vi "RelayController.vi"() -> ()   [LabVIEW 2016]
uses:
  <vilib>/Utility/miscctls.llb/LVRowAndColumnTypeDef.ctl
  <vilib>/Utility/file.llb/Read Delimited Spreadsheet (string).vi
  <vilib>/Utility/file.llb/Write Delimited Spreadsheet (string).vi
panel:
  out "running?":bool
  out "Controller OK?":bool
  out "countdown":dbl
  in  "resolution (ms)":u32=100 min=100 max=1000
  out "relay message":string
  in  "Port Name":refnum<visa-resource-name>
  in  "save sequence":bool
  in  "start seq":bool
  in  "Delete":bool
  in  "Insert":bool
  in  "Duration (s)":dbl=30.0
  in  "Set to OFF #":string
  in  "Set to ON #":string
  in  "Seq#":u32
  out "Sequence list":string[][](table)
  in  "load sequence":bool
  out "Current time":timestamp format="%<%.3X %x>T"
  out "Relay 24-31":bool[](array[boolean])
  out "Relay 8-15":bool[](array[boolean])
  out "Relay 16-23":bool[](array[boolean])
  in  "quit":bool
  in  "Typical duration (s)":dbl=30.0 min=0.0
  out "Relay 0-7":bool[](array[boolean])
  # "0"
  # "1"
  # "2"
  # "3"
  # "4"
  # "5"
  # "6"
  # "7"
  # "8"
  # "9"
  # "10"
  # "11"
  # "12"
  # "13"
  # "14"
  # "15"
  # "16"
  # "17"
  # "18"
  # "19"
  # "20"
  # "21"
  # "22"
  # "23"
  # "24"
  # "25"
  # "26"
  # "27"
  # "28"
  # "29"
  # "30"
  # "31"
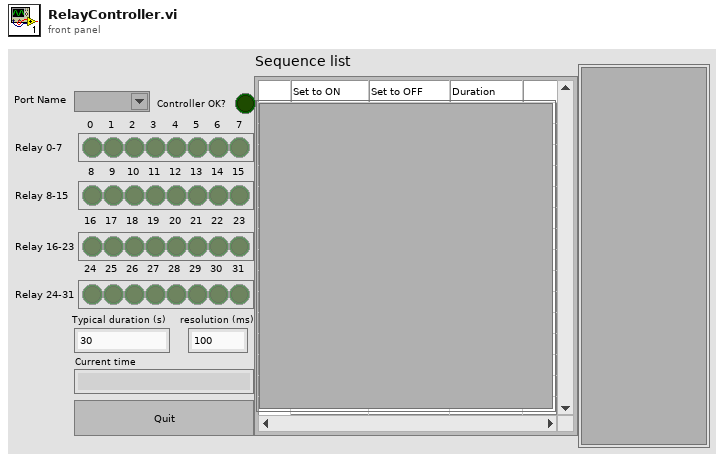
[diagram p1: front panel]
types:
  T1 = enum8{"Enabled", "Disabled", "Disabled and Grayed Out"}
  T2 = cluster{"Set to ON":string, "Set to OFF":string, "Duration (s)":dbl}[]
  T3 = cluster{"baud rate (9600)":u32, "data bits (8)":u16, "stop bits (10: 1 bit)":u16, "parity (0:none)":enum16{"None", "Odd", "Even", "Mark", "Space"}, "flow control (0:none)":u16, "timeout (10sec)":u32, "Enable Termination\nChar (T)":bool, "termination char\n(0xA = '\\n' = LF)\n(0xD = '\\r' = CF) ":u8}
  T4 = typedef "LVRowAndColumnTypeDef.ctl" = cluster{"Row":i32, "Column":i32}
  T5 = cluster{"Set to ON":string, "Set to OFF":string, "Duration (s)":dbl}
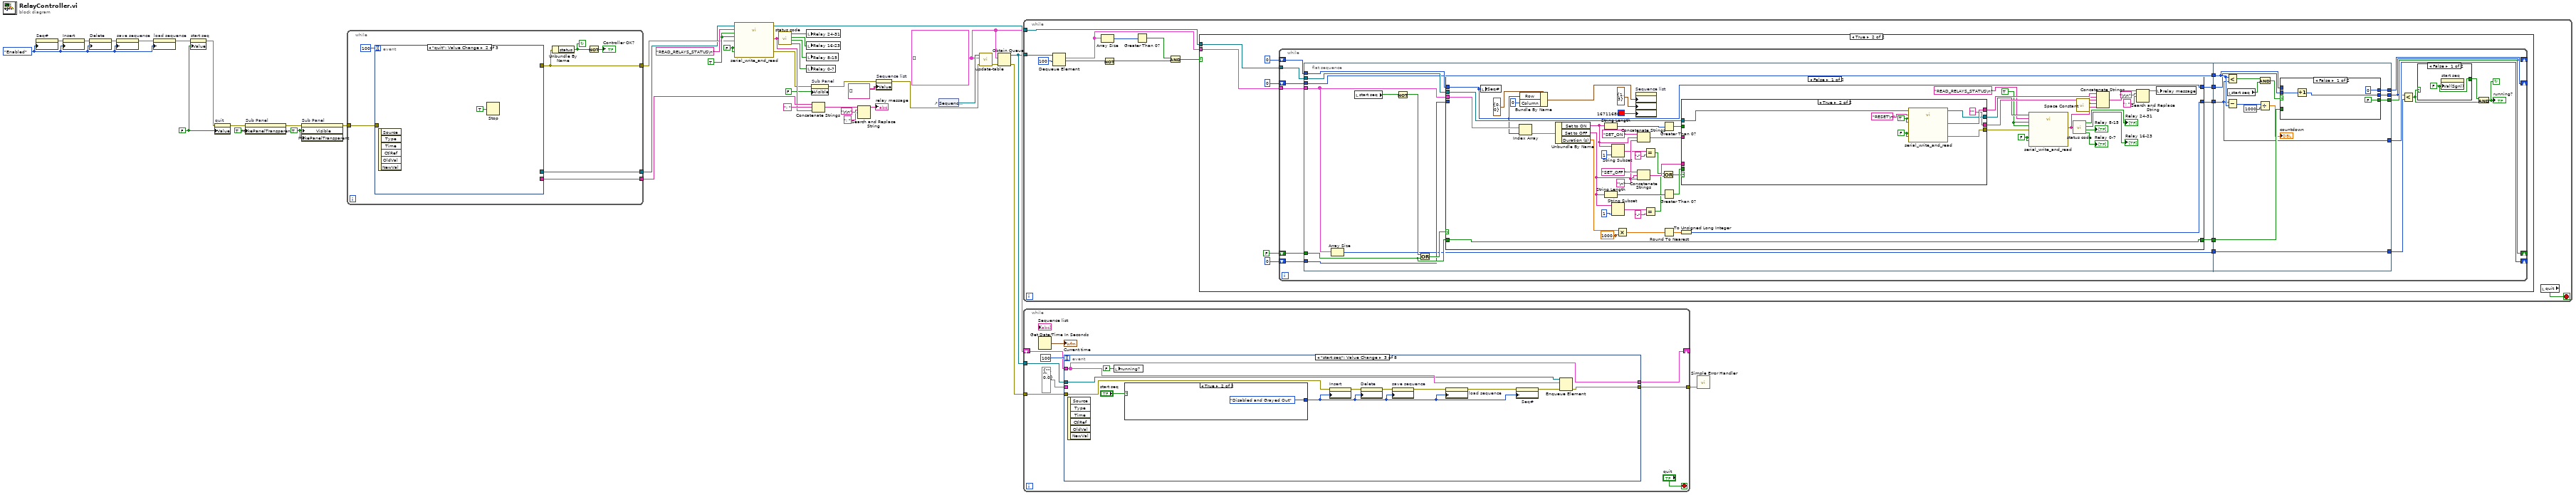
[diagram p0: block diagram]
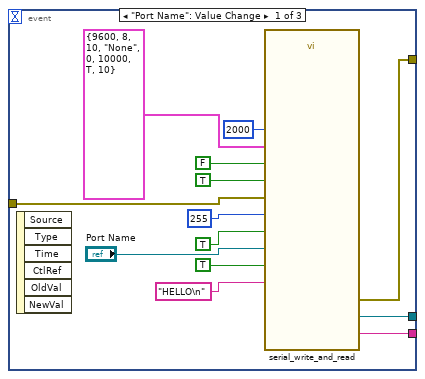
[diagram p2: hidden frame]
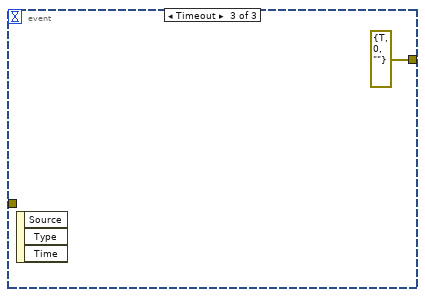
[diagram p3: hidden frame]
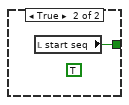
[diagram p5: hidden frame]
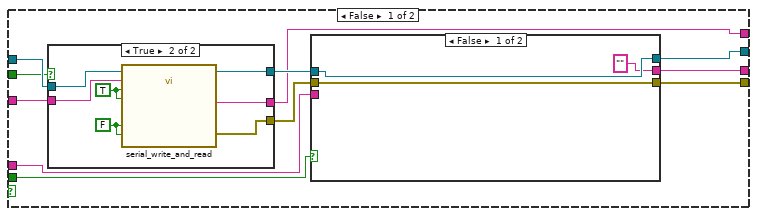
[diagram p6: hidden frame]
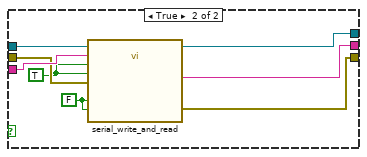
[diagram p7: hidden frame]
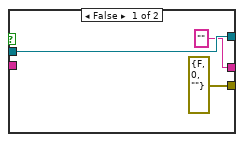
[diagram p8: hidden frame]
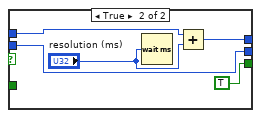
[diagram p10: hidden frame]
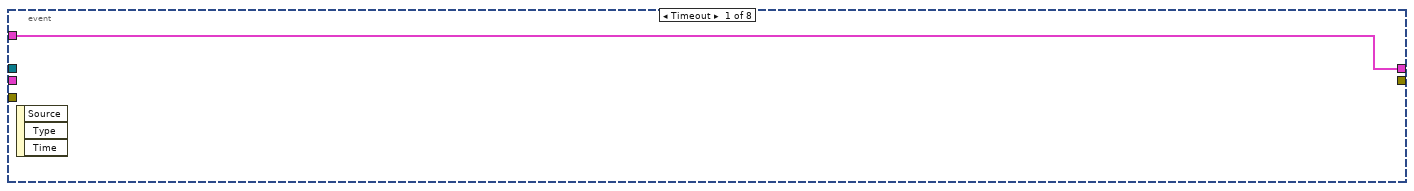
[diagram p11: hidden frame]
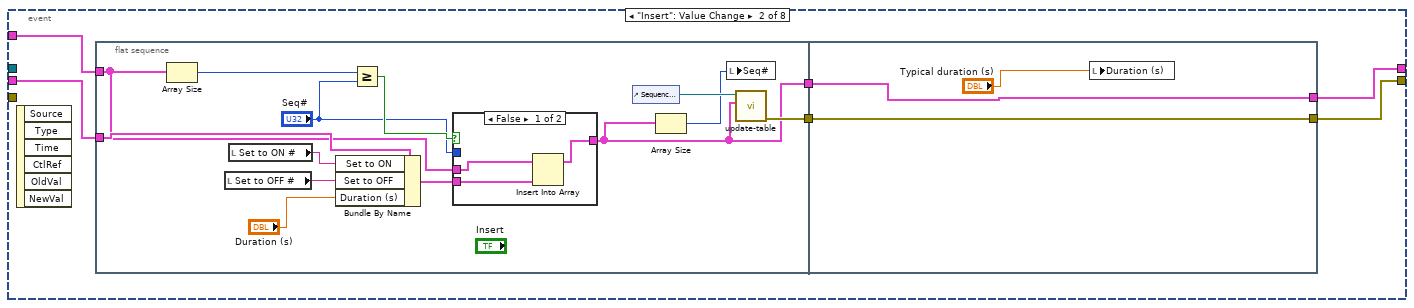
[diagram p12: hidden frame]
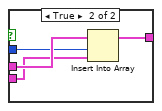
[diagram p13: hidden frame]
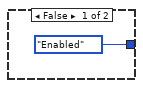
[diagram p14: hidden frame]
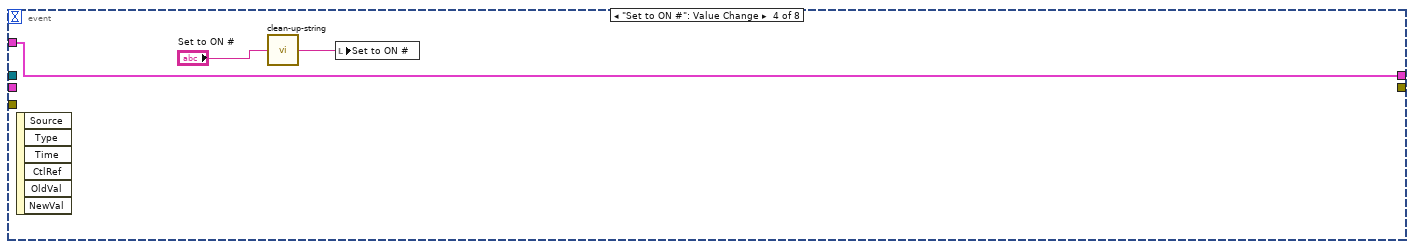
[diagram p15: hidden frame]
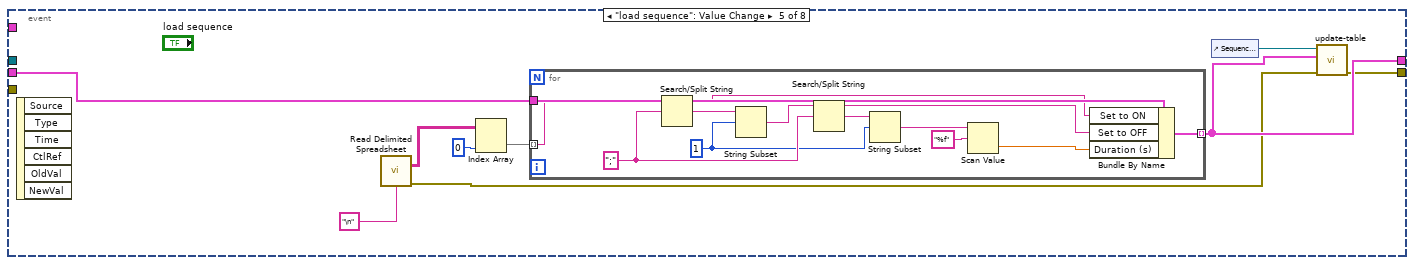
[diagram p16: hidden frame]
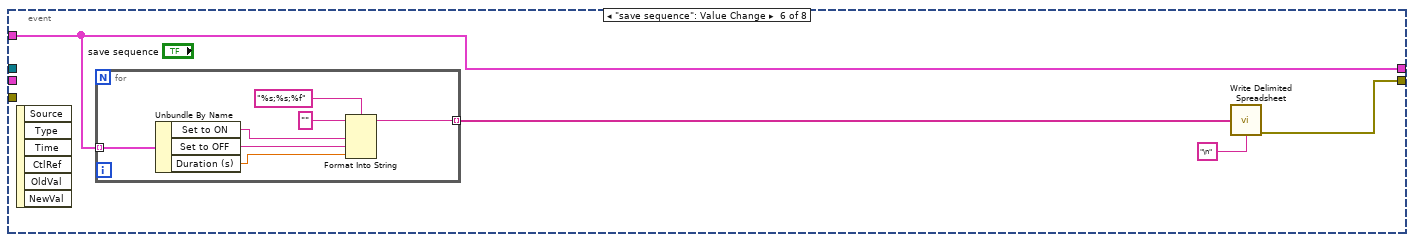
[diagram p17: hidden frame]
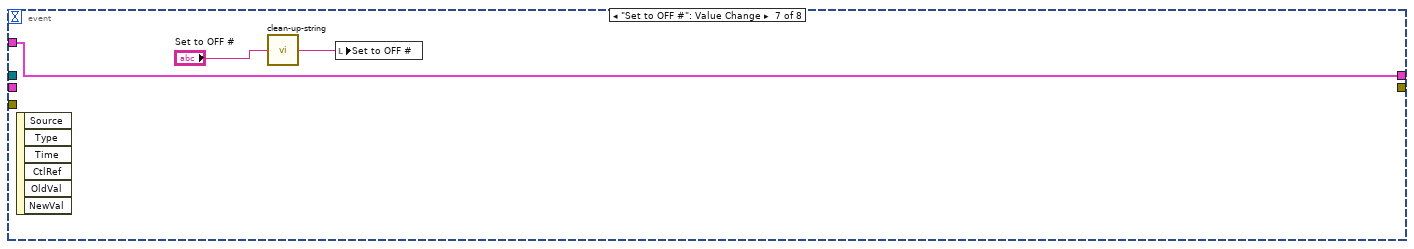
[diagram p18: hidden frame]
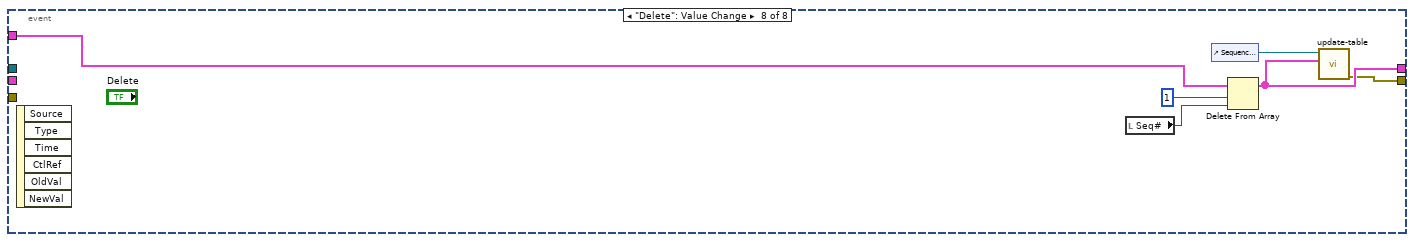
[diagram p19: hidden frame]
diagram:
  w6 = TRUE ("Visible")
  w27 = FALSE ("reconnect?")
  w28 = TRUE
  w13 = T1."Enabled" ("Disabled")
  w34 = FALSE ("start seq")
  w37 = T2 []
  n1 = property on="Seq#" class="DigNum (strict)"("DisabledEnum"=w13) -> (error out=w14:errorcluster)  [unwired: 2 in, 1 out]
  n2 = property on="Insert" class="Bool"(error in=w14, "DisabledEnum"=w13) -> (error out=w33:errorcluster)  [unwired: 1 in, 1 out]
  n3 = property on="Delete" class="Bool"(error in=w33, "DisabledEnum"=w13) -> (error out=w32:errorcluster)  [unwired: 1 in, 1 out]
  n4 = property on="save sequence" class="Bool"(error in=w32, "DisabledEnum"=w13) -> (error out=w31:errorcluster)  [unwired: 1 in, 1 out]
  n5 = property on="load sequence" class="Bool"(error in=w31, "DisabledEnum"=w13) -> (error out=w30:errorcluster)  [unwired: 1 in, 1 out]
  n6 = property on="start seq" class="Bool (strict)"(error in=w30, "Value"=w34) -> (error out=w35:errorcluster)  [unwired: 1 in, 1 out]
  n7 = property on="quit" class="Bool (strict)"(error in=w35, "Value"=w34) -> (error out=w12:errorcluster)  [unwired: 1 in, 1 out]
  n8 = property on="Sub Panel" class="SubPnl"(error in=w12, "MakePanelTransparent"=TRUE ("Panel Transparent")) -> (error out=w5:errorcluster)  [unwired: 1 in, 1 out]
  n9 = property on="Sub Panel" class="SubPnl"(error in=w5, "Visible"=w6, "MakePanelTransparent"=w6) -> (error out=w4:errorcluster)  [unwired: 1 in, 1 out]
  n10 = while {
    tunnel: [w48] -> w8
    tunnel: [w47] -> w23
    tunnel: w4 -> [w46]
    tunnel: [w45] -> w24
    stop <- w43 continue-if-true
    n11 = event shown="[1] \"quit\": Value Change" {
      selector: _ -> [_ _ _]
      dyn-events: _ -> [_ _ _]
      timeout: 100 -> [_ _ _]
      tunnel: [w54 _ _] -> w48
      tunnel: w46 -> [w51 _ _]
      tunnel: [w50 _ errorcluster {"status"=TRUE, "code"=0, "source"=""} ("error out")] -> w45
      tunnel: [w49 _ _] -> w47
      event "Port Name": Value Change {
        n12 = event-data() -> ()  [unwired: 1 in, 6 out]
        n13 = call "serial_write_and_read.vi"("port name in"="Port Name", "reconnect?"=TRUE, "disconnect?"=FALSE, "write buffer"="HELLO\n", "do writing?"=TRUE, "expecting response?"=TRUE, "error in"=w51, "expected max length"=u32 255, "connection parameters"=T3 {"baud rate (9600)"=9600, "data bits (8)"=8, "stop bits (10: 1 bit)"=10, "parity (0:none)"=enum."None", "flow control (0:none)"=0, "timeout (10sec)"=10000, "Enable Termination\nChar (T)"=TRUE, "termination char\n(0xA = '\\n' = LF)\n(0xD = '\\r' = CF) "=10}, "COM response delay"=u32 2000) -> ("port name out"=w54:refnum<visa-resource-name>, "read buffer"=w49:string, "error out"=w50:errorcluster)  [unwired: 3 in]
      }
      event "quit": Value Change {
        n14 = event-data() -> ()  [unwired: 1 in, 6 out]
        n15 = Stop(stop? (T)=TRUE) -> ()
      }
      event Timeout {
        n16 = event-data() -> ()  [unwired: 1 in, 3 out]
      }
    }
    n17 = Unbundle By Name(w45) -> ("status"=w43:bool)
    n18 = Not(x=w43) -> (.not. x?=→"Controller OK?":bool)
  }
  n19 = call "serial_write_and_read.vi"("port name in"=w8, "reconnect?"=w27, "disconnect?"=w27, "write buffer"="READ_RELAYS_STATUS\n", "do writing?"=w28, "expecting response?"=w28, "error in"=w24) -> ("port name out"=w7:refnum<visa-resource-name>, "read buffer"=w21:string, "error out"=w3:errorcluster)  [unwired: 6 in]
  n20 = call "status code.vi"("status code"=w21) -> ("Relay 24-31"=w15:bool[], "Relay 16-23"=w16:bool[], "Relay 8-15"=w17:bool[], "Relay 0-7"=w18:bool[])
  n21 = local write "Relay 24-31"(w15) -> ()
  n22 = local write "Relay 16-23"(w16) -> ()
  n23 = local write "Relay 8-15"(w17) -> ()
  n24 = local write "Relay 0-7"(w18) -> ()
  n25 = property on="Sub Panel" class="SubPnl"(error in=w3, "Visible"=FALSE) -> (error out=w2:errorcluster)  [unwired: 1 in, 1 out]
  n26 = Concatenate Strings(w23, "; " ("string"), w21) -> (w20:string)
  n27 = Search and Replace String(input string=w20, search string="\r\n", replace string="; " ("replace string (\"\")")) -> (result string=→"relay message":string)  [unwired: 5 in, 3 out]
  n28 = property on="Sequence list" class="Tbl (strict)"(error in=w2, "Value"=string[][] []) -> (error out=w11:errorcluster)  [unwired: 1 in, 1 out]
  n29 = control-ref of="Sequence list"() -> (w39:refnum<vi>)
  n30 = call "update-table.vi"("error in (no error)"=w11, "contents"=w37, "Table ref in"=w39) -> ("error out"=w10:errorcluster)  [unwired: 3 in, 1 out]
  n31 = Obtain Queue(element data type=w37, error in (no error)=w10) -> (queue out=w36:refnum<queue>, error out=w9:errorcluster)  [unwired: 3 in, 1 out]
  n32 = while {
    tunnel: w36 -> [w73]
    tunnel: w7 -> [w65]
    stop <- w64 stop-if-true
    n33 = Dequeue Element(queue=w73, timeout in ms (-1)=100) -> (element=w71:T2, timed out?=w69:bool)  [unwired: 1 in, 2 out]
    n34 = Array Size(array=w71) -> (size(s)=w70:i32)
    n35 = Not(x=w69) -> (.not. x?=w67:bool)
    n36 = Greater Than 0?(x=w70) -> (x > 0?=w68:bool)
    n37 = And(x=w68, y=w67) -> (x .and. y?=w66:bool)
    n38 = case shown="True" w66 {
      tunnel: w71 -> [_ w79]
      tunnel: w65 -> [_ w75]
      frame False {
      }
      frame True {
        n39 = while {
          tunnel: w79 -> [w90]
          shift-right: [w93] -> _
          shift-left: u32 0 -> [w87]
          shift-right: [w81] -> _
          shift-left: 0 -> [w82]
          shift-right: [w96] -> _
          shift-left: FALSE -> [w98]
          tunnel: w75 -> [w97]
          shift-right: [w83] -> _
          shift-left: u32 0 -> [w89]
          stop <- w80 continue-if-true
          n40 = flat-sequence {
            tunnel: w98 -> [w107]
            tunnel: w97 -> [w113]
            tunnel: w82 -> [w106]
            tunnel: [w112] -> w95
            tunnel: [w111] -> w94
            tunnel: w90 -> [w101]
            tunnel: w89 -> [w104]
            tunnel: [w105] -> w88
            tunnel: w87 -> [w103]
            tunnel: [w103] -> w86
            tunnel: [w102] -> w85
            tunnel: [w209] -> w81
            tunnel: [w217] -> w96
            tunnel: w95 -> [w218]
            tunnel: w94 -> [w210]
            tunnel: [w222] -> w93
            tunnel: w88 -> [w211]
            tunnel: w86 -> [w213]
            tunnel: w85 -> [w212]
            tunnel: [w212] -> w84
            tunnel: [w211] -> w83
            frame #0 {
              n41 = Array Size(array=w101) -> (size(s)=w102:i32)
              n42 = local read "start seq"() -> (w110:bool)
              n43 = Not(x=w110) -> (.not. x?=w109:bool)
              n44 = Or(x=w109, y=w107) -> (x .or. y?=w108:bool)
              n45 = case shown="False" w108 {
                tunnel: w113 -> [w165 _]
                tunnel: [w133 w207] -> w112
                tunnel: w106 -> [w114 w208]
                tunnel: [w114 w208] -> w111
                tunnel: w107 -> [w133 w207]
                tunnel: [w119 w206] -> w105
                tunnel: w104 -> [_ w206]
                tunnel: w101 -> [w122 _]
                frame False {
                  w134 = FALSE ("reconnect?")
                  w135 = TRUE
                  w150 = "\n" ("string")
                  n46 = local write "Seq#"(w114) -> ()
                  n47 = Index Array(array=w122, index=w114) -> (element=w127:T5)
                  n48 = Bundle By Name(cluster=T4 {"Row"=0, "Column"=0} ("Selection Start"), "Row"=w114, "Column"=0) -> (w131:T4)
                  n49 = Unbundle By Name(w127) -> ("Set to ON"=w121:string, "Set to OFF"=w120:string, "Duration (s)"=w126:dbl)
                  n50 = String Length(string=w121) -> (length=w148:i32)
                  n51 = String Length(string=w120) -> (length=w147:i32)
                  n52 = String Subset(string=w121, length (rest)=1 ("length (rest)")) -> (substring=w142:string)  [unwired: 1 in]
                  n53 = String Subset(string=w120, length (rest)=1 ("length (rest)")) -> (substring=w139:string)  [unwired: 1 in]
                  n54 = Multiply(x=w126, y=1000.0) -> (x*y=w124:dbl)
                  n55 = property on="Sequence list" class="Tbl (strict)"("Selection Start"=w131, "Selection Size"=T4 {"Row"=1, "Column"=3}, "Selection Color"=u32 16711680) -> ()  [unwired: 2 in, 2 out]
                  n56 = Concatenate Strings("SET_ON " ("string"), w121, w150) -> (w163:string)
                  n57 = Concatenate Strings("SET_OFF " ("string"), w120, w150) -> (w161:string)
                  n58 = Equal?(x=w142, y="-") -> (x = y?=w138:bool)
                  n59 = Equal?(x=w139, y="-") -> (x = y?=w137:bool)
                  n60 = Or(x=w138, y=w137) -> (x .or. y?=w136:bool)
                  n61 = Greater Than 0?(x=w148) -> (x > 0?=w146:bool)
                  n62 = Greater Than 0?(x=w147) -> (x > 0?=w145:bool)
                  n63 = Round To Nearest(number=w124) -> (nearest integer value=w123:dbl)
                  n64 = To Unsigned Long Integer(number=w123) -> (unsigned 32bit integer=w119:u32)
                  n65 = case shown="True" w136 {
                    tunnel: w165 -> [w176 w204]
                    tunnel: w163 -> [w175 _]
                    tunnel: w161 -> [w174 _]
                    tunnel: [w172 w203] -> w160
                    tunnel: [w171 "" ("read buffer")] -> w159
                    tunnel: [w170 w200] -> w157
                    tunnel: [w168 w199] -> w149
                    tunnel: w146 -> [w167 _]
                    tunnel: w145 -> [w166 _]
                    frame False {
                      n66 = case shown="True" w167 {
                        tunnel: w176 -> [w190 w197]
                        tunnel: w175 -> [_ w196]
                        tunnel: [w190 w195] -> w173
                        tunnel: ["" ("read buffer") w194] -> w172
                        tunnel: [errorcluster {"status"=FALSE, "code"=0, "source"=""} ("error out") w193] -> w169
                        frame False {
                        }
                        frame True {
                          w191 = FALSE ("reconnect?")
                          w192 = TRUE ("do writing?")
                          n67 = call "serial_write_and_read.vi"("port name in"=w197, "reconnect?"=w191, "disconnect?"=w191, "write buffer"=w196, "do writing?"=w192, "expecting response?"=w192) -> ("port name out"=w195:refnum<visa-resource-name>, "read buffer"=w194:string, "error out"=w193:errorcluster)  [unwired: 7 in]
                        }
                      }
                      n68 = case shown="False" w166 {
                        tunnel: w174 -> [_ w187]
                        tunnel: w173 -> [w179 w186]
                        tunnel: ["" ("read buffer") w185] -> w171
                        tunnel: [w179 w184] -> w170
                        tunnel: w169 -> [w177 w183]
                        tunnel: [w177 w182] -> w168
                        frame False {
                        }
                        frame True {
                          w180 = FALSE ("reconnect?")
                          w181 = TRUE
                          n69 = call "serial_write_and_read.vi"("port name in"=w186, "reconnect?"=w180, "disconnect?"=w180, "write buffer"=w187, "do writing?"=w181, "expecting response?"=w181, "error in"=w183) -> ("port name out"=w184:refnum<visa-resource-name>, "read buffer"=w185:string, "error out"=w182:errorcluster)  [unwired: 6 in]
                        }
                      }
                    }
                    frame True {
                      w201 = TRUE ("do writing?")
                      w202 = FALSE ("reconnect?")
                      n70 = call "serial_write_and_read.vi"("port name in"=w204, "reconnect?"=w202, "disconnect?"=w202, "write buffer"="RESET\n", "do writing?"=w201, "expecting response?"=w201) -> ("port name out"=w200:refnum<visa-resource-name>, "read buffer"=w203:string, "error out"=w199:errorcluster)  [unwired: 7 in]
                    }
                  }
                  n71 = call "serial_write_and_read.vi"("port name in"=w157, "reconnect?"=w134, "disconnect?"=w134, "write buffer"="READ_RELAYS_STATUS\n", "do writing?"=w135, "expecting response?"=w135, "error in"=w149) -> ("read buffer"=w155:string)  [unwired: 6 in, 2 out]
                  n72 = call "status code.vi"("status code"=w155) -> ("Relay 24-31"=→"Relay 24-31":bool[], "Relay 16-23"=→"Relay 16-23":bool[], "Relay 8-15"=→"Relay 8-15":bool[], "Relay 0-7"=→"Relay 0-7":bool[])
                  n73 = call <vilib>:"Space Constant.vi"() -> ("String"=w158:string)
                  n74 = Concatenate Strings(w160, w158, w159, w158, w155) -> (w118:string)
                  n75 = Search and Replace String(input string=w118, search string="\r\n", replace string="; " ("replace string (\"\")")) -> (result string=w115:string)  [unwired: 5 in, 3 out]
                  n76 = local write "relay message"(w115) -> ()
                }
                frame True {
                }
              }
            }
            frame #1 {
              n77 = Less?(x=w213, y=w211) -> (x < y?=w220:bool)
              n78 = Subtract(x=w211, y=w213) -> (x-y=w216:u32)
              n79 = local read "start seq"() -> (w221:bool)
              n80 = Divide(x=w216, y=u32 1000) -> (x/y=→"countdown":dbl)
              n81 = And(x=w220, y=w221) -> (x .and. y?=w219:bool)
              n82 = case shown="False" w219 {
                tunnel: w213 -> [_ w231]
                tunnel: [u32 0 w230] -> w222
                tunnel: w218 -> [_ _]
                tunnel: [FALSE ("do writing?") TRUE ("do writing?")] -> w217
                tunnel: w210 -> [w224 w227]
                tunnel: [w223 w227] -> w209
                frame False {
                  n83 = Increment(x=w224) -> (x+1=w223:i32)
                }
                frame True {
                  n84 = Wait (ms)(milliseconds to wait="resolution (ms)") -> ()  [unwired: 1 out]
                  n85 = Add(x=w231, y="resolution (ms)") -> (x+y=w230:u32)
                }
              }
            }
          }
          n86 = Less?(x=w81, y=w84) -> (x < y?=w92:bool)
          n87 = case shown="False" w92 {
            tunnel: [w99 w100] -> w91
            frame False {
              w99 = FALSE ("start seq")
              n88 = property on="start seq" class="Bool (strict)"("Val(Sgnl)"=w99) -> ()  [unwired: 2 in, 2 out]
            }
            frame True {
              (unwired) TRUE ("running?")
              n89 = local read "start seq"() -> (w100:bool)
            }
          }
          n90 = And(x=w91, y=w92) -> (x .and. y?=w80:bool)
          "running?" <- w80
        }
      }
    }
    n91 = local read "quit"() -> (w64:bool)
  }
  n92 = while {
    shift-right: [w236] -> _
    shift-left: w37 -> [w238]
    tunnel: [w234] -> w40
    tunnel: w9 -> [w233]
    tunnel: w36 -> [w232]
    stop <- "quit" stop-if-true
    n93 = Get Date/Time In Seconds() -> (seconds since 1Jan1904=→"Current time":timestamp)
    n94 = event shown="[2] \"start seq\": Value Change" {
      selector: _ -> [_ _ _ _ _ _ _ _]
      dyn-events: _ -> [_ _ _ _ _ _ _ _]
      timeout: 100 -> [_ _ _ _ _ _ _ _]
      tunnel: w238 -> [w241 w246 w277 w285 _ w313 w321 w329]
      tunnel: T5 {"Set to ON"="", "Set to OFF"="", "Duration (s)"=0.0} ("element") -> [_ w247 _ _ w296 _ _ _]
      tunnel: [w241 w244 w277 w285 w290 w313 w321 w326] -> w236
      tunnel: [_ w245 w275 _ w289 w310 _ w324] -> w234
      tunnel: w233 -> [_ _ w281 _ _ _ _ _]
      tunnel: w232 -> [_ _ w276 _ _ _ _ _]
      event Timeout {
        n95 = event-data() -> ()  [unwired: 1 in, 3 out]
      }
      event "Insert": Value Change {
        n96 = event-data() -> ()  [unwired: 1 in, 6 out]
        n97 = flat-sequence {
          tunnel: w247 -> [w260]
          tunnel: w246 -> [w253]
          tunnel: [w250] -> w243
          tunnel: [w249] -> w242
          tunnel: [w269] -> w244
          tunnel: [w270] -> w245
          tunnel: w243 -> [w270]
          tunnel: w242 -> [w269]
          frame #0 {
            n98 = Array Size(array=w253) -> (size(s)=w255:i32)
            n99 = local read "Set to OFF #"() -> (w258:string)
            n100 = local read "Set to ON #"() -> (w259:string)
            n101 = Bundle By Name(cluster=w260, "Set to ON"=w259, "Set to OFF"=w258, "Duration (s)"="Duration (s)") -> (w251:T5)
            n102 = Greater Or Equal?(x=w255, y="Seq#") -> (x >= y?=w254:bool)
            n103 = case shown="False" w254 {
              tunnel: w253 -> [w263 w267]
              tunnel: "Seq#" -> [_ w266]
              tunnel: w251 -> [w262 w265]
              tunnel: [w261 w264] -> w249
              frame False {
                n104 = Insert Into Array(array=w263, new element=w262) -> (w261:T2)  [unwired: 1 in]
              }
              frame True {
                n105 = Insert Into Array(array=w267, index=w266, new element=w265) -> (w264:T2)
              }
            }
            n106 = control-ref of="Sequence list"() -> (w256:refnum<vi>)
            n107 = Array Size(array=w249) -> (size(s)=w248:i32)
            n108 = local write "Seq#"(w248) -> ()
            n109 = call "update-table.vi"("contents"=w249, "Table ref in"=w256) -> ("error out"=w250:errorcluster)  [unwired: 4 in, 1 out]
          }
          frame #1 {
            n110 = local write "Duration (s)"("Typical duration (s)") -> ()
          }
        }
      }
      event "start seq": Value Change {
        n111 = event-data() -> ()  [unwired: 1 in, 6 out]
        n112 = local write "running?"(FALSE ("running?")) -> ()
        n113 = case shown="True" "start seq" {
          tunnel: [T1."Enabled" ("Disabled") T1."Disabled and Grayed Out" ("Disabled")] -> w272
          frame False {
          }
          frame True {
          }
        }
        n114 = property on="Insert" class="Bool"(error in=w281, "DisabledEnum"=w272) -> (error out=w280:errorcluster)  [unwired: 1 in, 1 out]
        n115 = property on="Delete" class="Bool"(error in=w280, "DisabledEnum"=w272) -> (error out=w279:errorcluster)  [unwired: 1 in, 1 out]
        n116 = property on="save sequence" class="Bool"(error in=w279, "DisabledEnum"=w272) -> (error out=w278:errorcluster)  [unwired: 1 in, 1 out]
        n117 = property on="load sequence" class="Bool"(error in=w278, "DisabledEnum"=w272) -> (error out=w274:errorcluster)  [unwired: 1 in, 1 out]
        n118 = property on="Seq#" class="DigNum (strict)"(error in=w274, "DisabledEnum"=w272) -> (error out=w273:errorcluster)  [unwired: 1 in, 1 out]
        n119 = Enqueue Element(queue=w276, element=w277, error in (no error)=w273) -> (error out=w275:errorcluster)  [unwired: 1 in, 2 out]
      }
      event "Set to ON #": Value Change {
        n120 = event-data() -> ()  [unwired: 1 in, 6 out]
        n121 = call "clean-up-string.vi"("input string"="Set to ON #") -> ("string out"=w286:string)
        n122 = local write "Set to ON #"(w286) -> ()
      }
      event "load sequence": Value Change {
        n123 = event-data() -> ()  [unwired: 1 in, 6 out]
        n124 = call-poly <vilib>:"Read Delimited Spreadsheet.vi"("delimiter (\\t)"="\n" ("delimiter (\\t)")) -> ("all rows"=w294:string[][], "error out"=w288:errorcluster)  [unwired: 9 in, 4 out]
        n125 = Index Array(array=w294, index (col)=0 ("disabled index (col)")) -> (element=w292:string[])  [unwired: 1 in]
        n126 = for {
          tunnel: w296 -> [w309]
          tunnel: [w308] -> w290 mode=indexing
          tunnel: w292 -> [w306] mode=indexing
          w302 = 1 ("offset (0)")
          w303 = ";" ("search string/char (-)")
          n127 = Search/Split String(string=w306, search string/char (-)=w303) -> (substring before match=w299:string, match + rest of string=w305:string)  [unwired: 1 in, 1 out]
          n128 = String Subset(string=w305, offset (0)=w302) -> (substring=w304:string)  [unwired: 1 in]
          n129 = Search/Split String(string=w304, search string/char (-)=w303) -> (substring before match=w298:string, match + rest of string=w301:string)  [unwired: 1 in, 1 out]
          n130 = String Subset(string=w301, offset (0)=w302) -> (substring=w300:string)  [unwired: 1 in]
          n131 = Scan Value(string=w300, format string="%f") -> (value=w307:dbl)  [unwired: 1 in, 1 out]
          n132 = Bundle By Name(cluster=w309, "Set to ON"=w299, "Set to OFF"=w298, "Duration (s)"=w307) -> (w308:T5)
        }
        n133 = control-ref of="Sequence list"() -> (w291:refnum<vi>)
        n134 = call "update-table.vi"("error in (no error)"=w288, "contents"=w290, "Table ref in"=w291) -> ("error out"=w289:errorcluster)  [unwired: 3 in, 1 out]
      }
      event "save sequence": Value Change {
        n135 = event-data() -> ()  [unwired: 1 in, 6 out]
        n136 = for {
          tunnel: w313 -> [w320] mode=indexing
          tunnel: [w314] -> w311 mode=indexing
          n137 = Unbundle By Name(w320) -> ("Set to ON"=w318:string, "Set to OFF"=w317:string, "Duration (s)"=w316:dbl)
          n138 = Format Into String(format string="%s;%s;%f", initial string="", w318, w317, w316) -> (resulting string=w314:string)  [unwired: 1 in, 1 out]
        }
        n139 = call-poly <vilib>:"Write Delimited Spreadsheet.vi"("1D data"=w311, "delimiter (\\t)"="\n" ("delimiter (\\t)")) -> ("error out"=w310:errorcluster)  [unwired: 12 in, 1 out]
      }
      event "Set to OFF #": Value Change {
        n140 = event-data() -> ()  [unwired: 1 in, 6 out]
        n141 = call "clean-up-string.vi"("input string"="Set to OFF #") -> ("string out"=w322:string)
        n142 = local write "Set to OFF #"(w322) -> ()
      }
      event "Delete": Value Change {
        n143 = event-data() -> ()  [unwired: 1 in, 6 out]
        n144 = local read "Seq#"() -> (w328:u32)
        n145 = control-ref of="Sequence list"() -> (w325:refnum<vi>)
        n146 = Delete From Array(array=w329, length=1 ("index"), index=w328) -> (array with subset deleted=w326:T2)  [unwired: 1 out]
        n147 = call "update-table.vi"("contents"=w326, "Table ref in"=w325) -> ("error out"=w324:errorcluster)  [unwired: 4 in, 1 out]
      }
    }
  }
  n148 = call <vilib>:"Simple Error Handler.vi"("error in (no error)"=w40) -> ()  [unwired: 4 in, 5 out]
